vi "power_factors.vi"(9 "TauM":dbl[](array[numeric]) format="%10.4f", 10 "KappaM":dbl[](array[numeric]) format="%10.4e", 11 "RMESS":dbl[](array[numeric])) -> (1 "F_ch":dbl[](array[numeric]), 2 "tau_fact":dbl[](array[numeric]))   [LabVIEW 2014]
panel:
  out "U_eff":dbl[](array[numeric])
  out "beta":dbl[](array[numeric])
  out "g_C":dbl[](array[numeric])
  out "omega":dbl
  out "r_C":dbl=41.0
  out "U_0":dbl=5.0
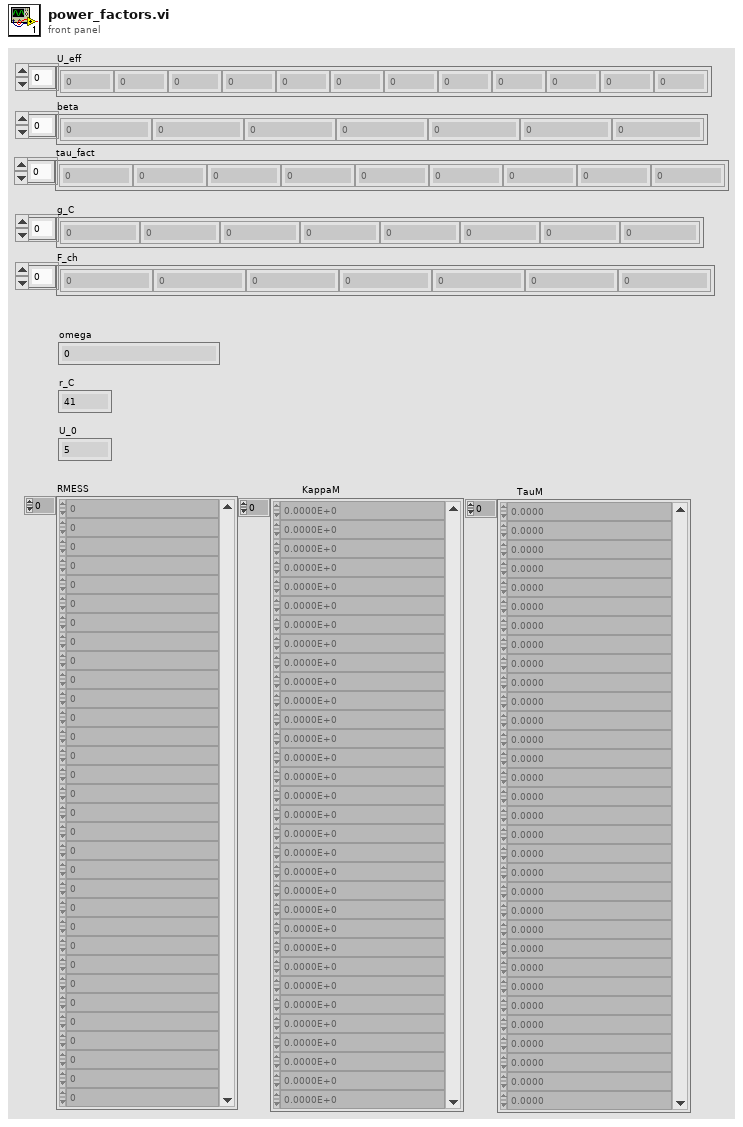
[diagram p1: front panel]
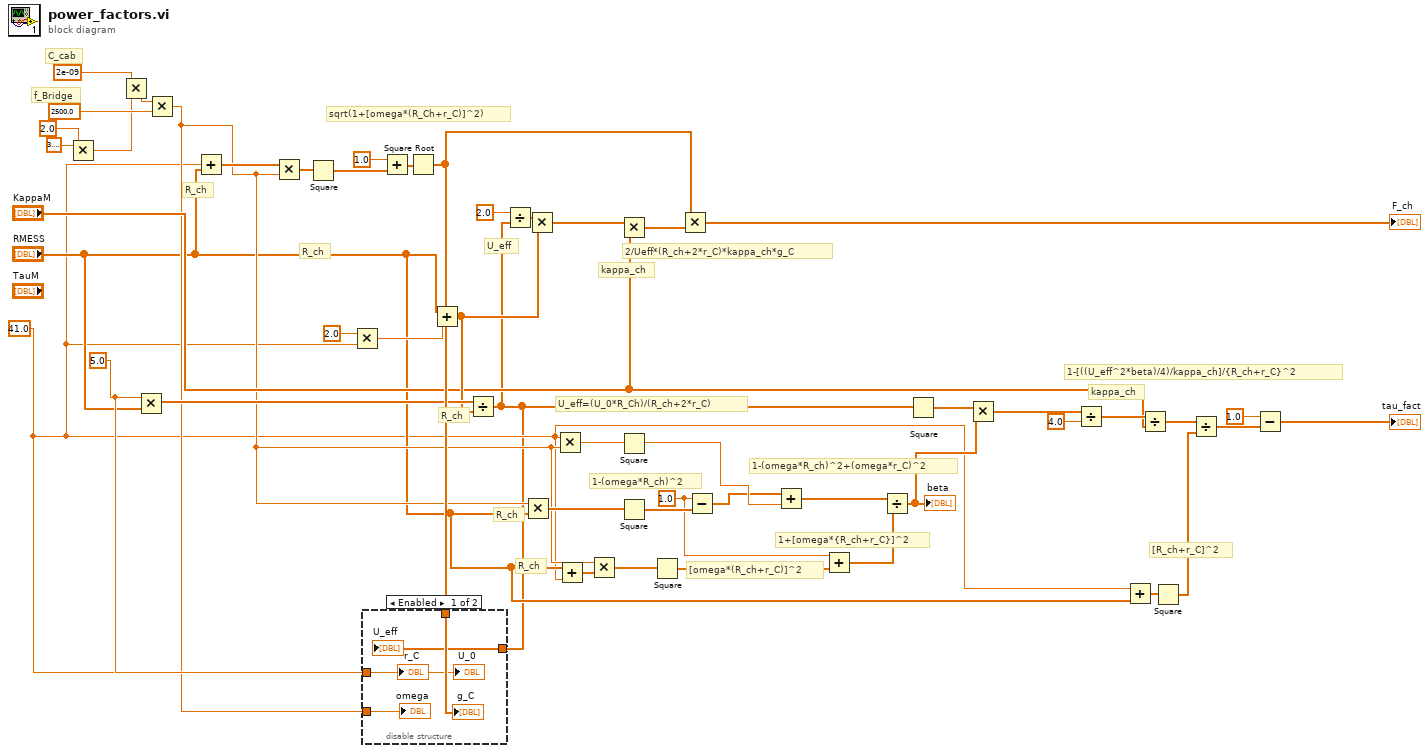
[diagram p0: block diagram]
diagram:
  w28 = 1.0 ("x")
  w35 = 5.0
  w2 = 41.0
  # "[R_ch+r_C]^2"
  # "[omega*(R_ch+r_C)]^2"
  # "U_eff"
  # "kappa_ch"
  # "kappa_ch"
  # "R_ch"
  # "R_ch"
  # "R_ch"
  # "R_ch"
  # "R_ch"
  # "1-[((U_eff^2*beta)/4)/kappa_ch]/{R_ch+r_C}^2"
  # "U_eff=(U_0*R_Ch)/(R_ch+2*r_C)"
  # "2/Ueff*(R_ch+2*r_C)*kappa_ch*g_C"
  # "sqrt(1+[omega*(R_Ch+r_C)]^2)"
  # "1+[omega*{R_ch+r_C}]^2"
  # "1-(omega*R_ch)^2+(omega*r_C)^2"
  # "1-(omega*R_ch)^2"
  # "C_cab"
  # "f_Bridge"
  n1 = Multiply(x=3.141592653589793, y=2.0) -> (x*y=w3:dbl)
  n2 = Multiply(x=2e-09, y=w3) -> (x*y=w48:dbl)
  n3 = Multiply(x=w35, y="RMESS") -> (x*y=w34:dbl[])
  n4 = Multiply(x=w48, y=2500.0) -> (x*y=w11:dbl)
  n5 = Add(x=w2, y="RMESS") -> (x+y=w12:dbl[])
  n6 = Multiply(x=w12, y=w11) -> (x*y=w13:dbl[])
  n7 = Square(x=w13) -> (x^2=w45:dbl[])
  n8 = Multiply(x=2.0, y=w2) -> (x*y=w41:dbl)
  n9 = Add(x=1.0, y=w45) -> (x+y=w44:dbl[])
  n10 = Square Root(x=w44) -> (sqrt(x)=w37:dbl[])
  n11 = Add(x="RMESS", y=w41) -> (x+y=w33:dbl[])
  n12 = Divide(x=w34, y=w33) -> (x/y=w1:dbl[])
  n13 = disable-structure shown="Enabled" {
    disable-tunnel: w37 -> [w54 _]
    disable-tunnel: w35 -> [w53 _]
    disable-tunnel: w11 -> [w52 _]
    disable-tunnel: w2 -> [w51 _]
    disable-tunnel: w1 -> [w50 _]
    frame Enabled {
      "omega" <- w52
      "r_C" <- w51
      "U_0" <- w53
      "g_C" <- w54
      "U_eff" <- w50
    }
    frame Disabled {
    }
  }
  n14 = Divide(x=2.0, y=w1) -> (x/y=w40:dbl[])
  n15 = Multiply(x=w11, y="RMESS") -> (x*y=w32:dbl[])
  n16 = Multiply(x=w40, y=w33) -> (x*y=w39:dbl[])
  n17 = Multiply(x=w2, y=w11) -> (x*y=w30:dbl)
  n18 = Add(x="RMESS", y=w2) -> (x+y=w27:dbl[])
  n19 = Multiply(x=w11, y=w27) -> (x*y=w26:dbl[])
  n20 = Multiply(x=w39, y="KappaM") -> (x*y=w38:dbl[])
  n21 = Square(x=w30) -> (x^2=w7:dbl)
  n22 = Square(x=w32) -> (x^2=w31:dbl[])
  n23 = Square(x=w26) -> (x^2=w18:dbl[])
  n24 = Multiply(x=w37, y=w38) -> (x*y=→"F_ch":dbl[])
  n25 = Subtract(x=w28, y=w31) -> (x-y=w6:dbl[])
  n26 = Add(x=w6, y=w7) -> (x+y=w29:dbl[])
  n27 = Add(x=w28, y=w18) -> (x+y=w25:dbl[])
  n28 = Divide(x=w29, y=w25) -> (x/y=w23:dbl[])
  "beta" <- w23
  n29 = Square(x=w1) -> (x^2=w24:dbl[])
  n30 = Multiply(x=w24, y=w23) -> (x*y=w17:dbl[])
  n31 = Divide(x=w17, y=4.0) -> (x/y=w21:dbl[])
  n32 = Add(x=w2, y="RMESS") -> (x+y=w9:dbl[])
  n33 = Divide(x=w21, y="KappaM") -> (x/y=w19:dbl[])
  n34 = Square(x=w9) -> (x^2=w10:dbl[])
  n35 = Divide(x=w19, y=w10) -> (x/y=w15:dbl[])
  n36 = Subtract(x=1.0, y=w15) -> (x-y=→"tau_fact":dbl[])
